vi "vartest.vi"(2 "consequencearray":T1(array[cluster])=[{"ling.var."="out", "x-min"=-1.0, "x-max"=1.0, "setarray"=[{"linguistic term"="NEo", "color"=0, "points"=[-1.0, -1.0000001192092896, -1.0000001192092896, 0.0]}, {"linguistic term"="ZEo", "color"=0, "points"=[-1.0000001192092896, 0.0, 0.0, 1.0000001192092896]}, {"linguistic term"="POo", "color"=0, "points"=[1.4901161193847656e-08, 1.0, 1.0, 1.0000001192092896]}]}] {"x-min" format="%.2f"; "x-max" format="%.2f"; "setarray"."points" min=-1.0 max=1.0 step=0.10000000149011612 format="%.2f"}, 3 "antecedancearray":T1(array[cluster])=[{"ling.var."="in1", "x-min"=-1.0, "x-max"=1.0, "setarray"=[{"linguistic term"="NE1", "color"=0, "points"=[-1.0, -1.0000001192092896, -1.0000001192092896, 0.0]}, {"linguistic term"="ZE1", "color"=0, "points"=[-1.0000001192092896, 0.0, 0.0, 1.0000001192092896]}, {"linguistic term"="PO1", "color"=0, "points"=[1.4901161193847656e-08, 1.0, 1.0, 1.0000001192092896]}]}, {"ling.var."="in2", "x-min"=-1.0, "x-max"=1.0, "setarray"=[{"linguistic term"="NE2", "color"=0, "points"=[-1.0, -1.0000001192092896, -1.0000001192092896, 0.0]}, {"linguistic term"="ZE2", "color"=0, "points"=[-1.0000001192092896, 0.0, 0.0, 1.0000001192092896]}, {"linguistic term"="PO2", "color"=0, "points"=[1.4901161193847656e-08, 1.0, 1.0, 1.0000001192092896]}]}, {"ling.var."="in3", "x-min"=-1.0, "x-max"=1.0, "setarray"=[{"linguistic term"="NE3", "color"=0, "points"=[-1.0, -1.0000001192092896, -1.0000001192092896, 0.0]}, {"linguistic term"="ZE3", "color"=0, "points"=[-1.0000001192092896, 0.0, 0.0, 1.0000001192092896]}, {"linguistic term"="PO3", "color"=0, "points"=[1.4901161193847656e-08, 1.0, 1.0, 1.0000001192092896]}]}, {"ling.var."="in4", "x-min"=-1.0, "x-max"=1.0, "setarray"=[{"linguistic term"="NE4", "color"=0, "points"=[-1.0, -1.0000001192092896, -1.0000001192092896, 0.0]}, {"linguistic term"="ZE4", "color"=0, "points"=[-1.0000001192092896, 0.0, 0.0, 1.0000001192092896]}, {"linguistic term"="PO4", "color"=0, "points"=[1.4901161193847656e-08, 1.0, 1.0, 1.0000001192092896]}]}] {"x-min" format="%.2f"; "x-max" format="%.2f"; "setarray"."points" min=-1.0 max=1.0 step=0.10000000149011612 format="%.2f"}) -> (0 "error out":errorcluster)   [LabVIEW 2017, in "NI_fuzzy logic.lvlib"]
doc: "Errorhandler VI for the Fuzzy-editors.\nGives out an errorcluster if the antecedance- or consequencearray isn«t OK.\n- more than 4 or no antecedancevariables\n- more than 1 or no consequencevariable\n- more than 9 or no terms in a variable"
uses:
  <vilib>/addons/control/fuzzy/NI_fuzzy logic.lvlib
panel:
  in  "no error":errorcluster
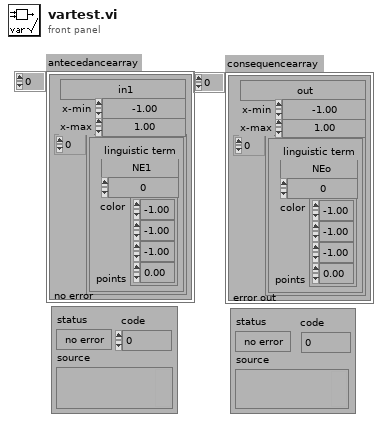
[diagram p1: front panel]
types:
  T1 = cluster{"ling.var.":string, "x-min":dbl, "x-max":dbl, "setarray":cluster{"linguistic term":string, "color":u32, "points":dbl[]}[]}[]
  T2 = cluster{"linguistic term":string, "color":u32, "points":dbl[]}[]
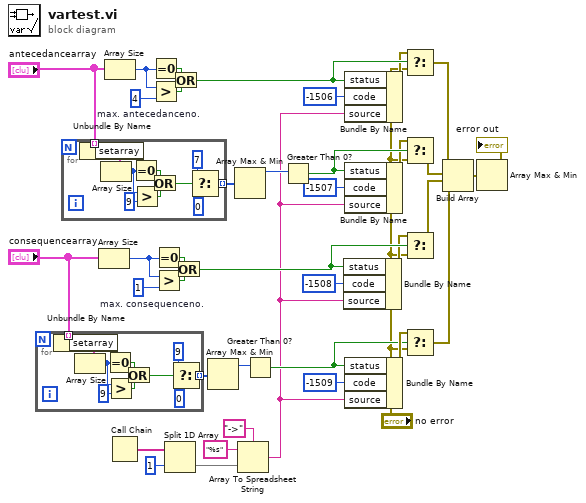
[diagram p0: block diagram]
diagram:
  w32 = 1  # max. consequenceno.
  w38 = 4  # max. antecedanceno.
  n1 = for {
    tunnel: "consequencearray" -> [w46] mode=indexing
    tunnel: [w47] -> w35 mode=indexing
    n2 = Unbundle By Name(w46) -> ("setarray"=w45:T2)
    n3 = Array Size(array=w45) -> (size(s)=w43:i32)
    n4 = Equal To 0?(x=w43) -> (x = 0?=w42:bool)
    n5 = Greater?(x=w43, y=9) -> (0:w41:bool)
    n6 = Or(x=w42, y=w41) -> (x .or. y?=w40:bool)
    n7 = Select(t=9, s=w40, f=0) -> (s? t:f=w47:i32)
  }
  n8 = for {
    tunnel: "antecedancearray" -> [w56] mode=indexing
    tunnel: [w57] -> w27 mode=indexing
    n9 = Unbundle By Name(w56) -> ("setarray"=w55:T2)
    n10 = Array Size(array=w55) -> (size(s)=w53:i32)
    n11 = Equal To 0?(x=w53) -> (x = 0?=w52:bool)
    n12 = Greater?(x=w53, y=9) -> (0:w51:bool)
    n13 = Or(x=w52, y=w51) -> (x .or. y?=w50:bool)
    n14 = Select(t=7, s=w50, f=0) -> (s? t:f=w57:i32)
  }
  n15 = Array Size(array="consequencearray") -> (size(s)=w31:i32)
  n16 = Array Size(array="antecedancearray") -> (size(s)=w39:i32)
  n17 = Call Chain() -> (call chain=w4:string[])
  n18 = Equal To 0?(x=w39) -> (x = 0?=w37:bool)
  n19 = Greater?(x=w39, y=w38) -> (0:w36:bool)
  n20 = Equal To 0?(x=w31) -> (x = 0?=w33:bool)
  n21 = Greater?(x=w31, y=w32) -> (0:w34:bool)
  n22 = Split 1D Array(array=w4, index=1) -> (second subarray=w2:string[])  [unwired: 1 out]
  n23 = Or(x=w37, y=w36) -> (x .or. y?=w24:bool)
  n24 = Or(x=w33, y=w34) -> (x .or. y?=w19:bool)
  n25 = Array Max & Min(array=w35) -> (max value=w30:i32)  [unwired: 3 out]
  n26 = Array Max & Min(array=w27) -> (max value=w11:i32)  [unwired: 3 out]
  n27 = Array To Spreadsheet String(delimiter (Tab)="->", array=w2, 3:"%s" ("format string")) -> (spreadsheet string=w1:string)
  n28 = Greater Than 0?(x=w30) -> (x > 0?=w16:bool)
  n29 = Greater Than 0?(x=w11) -> (x > 0?=w22:bool)
  n30 = Bundle By Name(cluster="no error", "status"=w19, "code"=-1508, "source"=w1) -> (w18:errorcluster)
  n31 = Bundle By Name(cluster="no error", "status"=w24, "code"=-1506, "source"=w1) -> (w23:errorcluster)
  n32 = Bundle By Name(cluster="no error", "status"=w22, "code"=-1507, "source"=w1) -> (w21:errorcluster)
  n33 = Bundle By Name(cluster="no error", "status"=w16, "code"=-1509, "source"=w1) -> (w17:errorcluster)
  n34 = Select(t=w23, s=w24, f="no error") -> (s? t:f=w25:errorcluster)
  n35 = Select(t=w21, s=w22, f="no error") -> (s? t:f=w20:errorcluster)
  n36 = Select(t=w18, s=w19, f="no error") -> (s? t:f=w14:errorcluster)
  n37 = Select(t=w17, s=w16, f="no error") -> (s? t:f=w13:errorcluster)
  n38 = Build Array(w25, w20, w14, w13) -> (w28:errorcluster[])
  n39 = Array Max & Min(array=w28) -> (max value=→"error out":errorcluster)  [unwired: 3 out]
